vi "DQMH_API_GetInstance.vi"(0 "reference in":refnum<class "DQMH_API.lvclass"> caption="This control should only be used when\na sub class is inheriting this class", 11 "error in (no error)":errorcluster) -> (3 "ObjectQueueName":string caption="This queue name could be used to destroy\nthe named queue that is used to hold the\nreference in the clean up.", 4 "reference out":refnum<class "DQMH_API.lvclass">, 6 "NewObjectCreated":bool, 10 "DVRRefOut":refnum<data-value>, 15 "error out":errorcluster)   [LabVIEW 2016, in "DQMH_API.lvclass"]
uses:
  <resource>/Framework/Providers/Open_GDS/UML/DQMH_API_class/DQMH_API.lvclass
  <resource>/Framework/Providers/Open_GDS/UML/DQMH_API_class/protected/ObjectAttributes.ctl
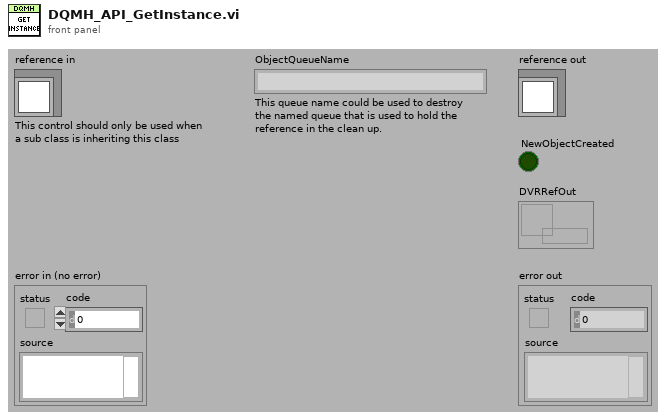
[diagram p1: front panel]
types:
  T1 = enum16{"Create or look up existing", "Look up existing"}
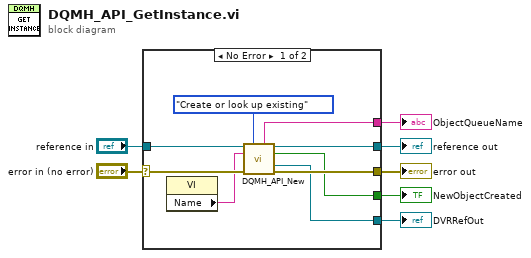
[diagram p0: block diagram]
diagram:
  n1 = case shown="No Error" "error in (no error)" {
    selector: "error in (no error)" -> [w15 w18]
    tunnel: [w16 w17] -> w7
    tunnel: [w14 w18] -> w5
    tunnel: "reference in" -> [w12 w17]
    tunnel: [w11 _] -> w3
    tunnel: [w10 _] -> w2
    tunnel: [w8 _] -> w1
    frame No Error {
      n2 = property class="VI"() -> ("Name"=w13:string)  [unwired: 2 in, 2 out]
      n3 = call <resource>:"DQMH_API_New.vi"("reference in"=w12, "CreateMethod(Create or look up existing)"=T1."Create or look up existing", "Object name"=w13, "error in (no error)"=w15) -> ("ObjectQueueName"=w8:string, "reference out"=w16:refnum<class "DQMH_API.lvclass">, "NewObjectCreated"=w11:bool, "DVRRefOut"=w10:refnum<data-value>, "error out"=w14:errorcluster)  [unwired: 7 in]
    }
    frame Error {
    }
  }
  "reference out" <- w7
  "error out" <- w5
  "NewObjectCreated" <- w3
  "DVRRefOut" <- w2
  "ObjectQueueName" <- w1
